vi "array -- bilinear regression 2D -- V2.vi"(7 "action":T2, 9 "fit map IN":map{T1, dbl}(c390), 11 "xyz IN":cluster{"x":dbl[], "y":dbl[], "z":dbl[]}={"x"=[0.0, 0.0, 0.0, -1.0, -1.0, -1.0, 1.0, 1.0, 1.0], "y"=[-1.0, 0.0, 1.0, -1.0, 0.0, 1.0, -1.0, 0.0, 1.0], "z"=[1.0, 0.0, 1.0, 4.0, 1.0, 0.0, 0.0, 1.0, 4.0]}) -> (1 "fit map out":map{T1, dbl}(c390), 3 "xyz OUT":cluster{"x":dbl[], "y":dbl[], "z":dbl[]}={"x"=[0.0, 0.0, 0.0, -1.0, -1.0, -1.0, 1.0, 1.0, 1.0], "y"=[-1.0, 0.0, 1.0, -1.0, 0.0, 1.0, -1.0, 0.0, 1.0], "z"=[1.0, 0.0, 1.0, 4.0, 1.0, 0.0, 0.0, 1.0, 4.0]})   [LabVIEW 2021]
uses:
  array -- fit control .ctl
  array -- bilinear regression 2D.ctl
  <vilib>/Analysis/baseanly.llb/Matrix Type of Inverse Matrix.ctl
  <vilib>/Analysis/baseanly.llb/Real A x B.vi
  <vilib>/Analysis/Matrix/Numeric/Conversions/Array To Matrix - RA2.vi
  <vilib>/Analysis/baseanly.llb/Real Inverse Matrix.vi
  <vilib>/Analysis/Matrix/Numeric/Conversions/Matrix To Array - RM.vi
  <vilib>/Analysis/NI_AALBase.lvlib
  <vilib>/Analysis/Matrix/NI_Matrix.lvlib
panel:
  out "y":dbl[](array[numeric])=[-1.0, 0.0, 1.0, -1.0, 0.0, 1.0, -1.0, 0.0, 1.0]
  out "fit  IN":dbl[](array[numeric])=[1.9, 2.6, 3.3, 1.0, 2.7, 3.9]
  out "fit OUT":dbl[](array[numeric])=[1.0, 1.0, 1.0, 0.0, 0.0, 0.0]
  out "z":dbl[](array[numeric])=[1.0, 0.0, 1.0, 4.0, 1.0, 0.0, 0.0, 1.0, 4.0]
  out "x":dbl[](array[numeric])=[0.0, 0.0, 0.0, -1.0, -1.0, -1.0, 1.0, 1.0, 1.0]
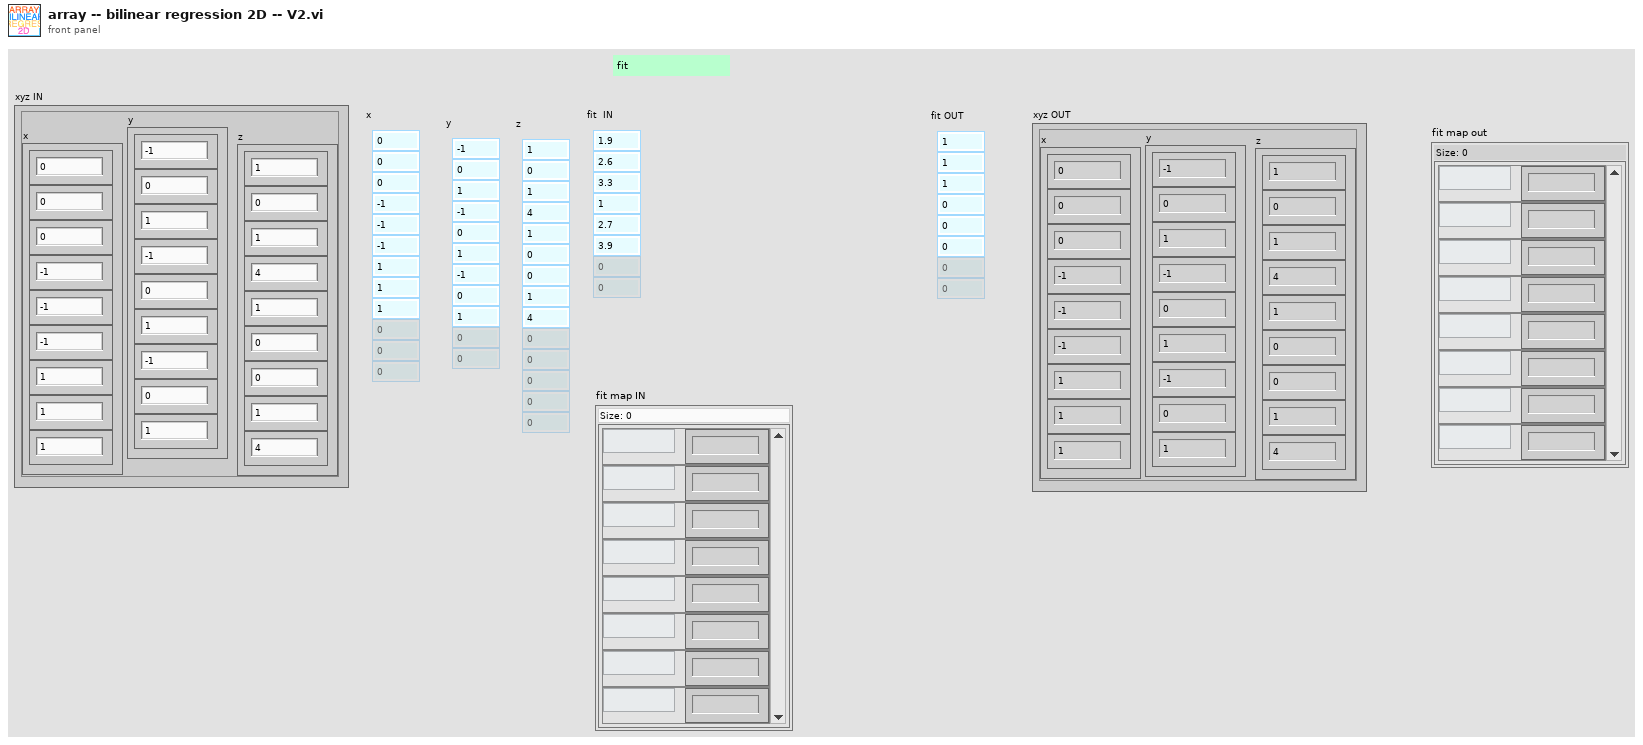
[diagram p1: front panel]
types:
  T1 = typedef "array -- bilinear regression 2D.ctl" = enum16{"1", "x", "y", "xx", "xy", "yy", "xxy", "xyy", "yyy", "xxx", "xxyy", "xyyy", "xxxy", "yyyy", "xxxx", "xxz", "xyz", "yyz", "xz", "yz", "z", "wwz", "ywz", "xwz", "xxxw", "xxyw", "xyyw", "yyyw", "xxww", "xyww", "yyww", "xwww", "ywww", "wwww", "ww", "xw", "yw", "w", "wz"}
  T2 = typedef "array -- fit control .ctl" = enum16{"fit", "calc", "check", "init"}
  T3 = typedef "NI_AALBase.lvlib/Matrix Type of Inverse Matrix.ctl" = enum32{"General", "Positive Definite", "Lower Triangular", "Upper Triangular"}
  T4 = typedef "NI_Matrix.lvlib/RealMatrix.ctl" = dbl[][]
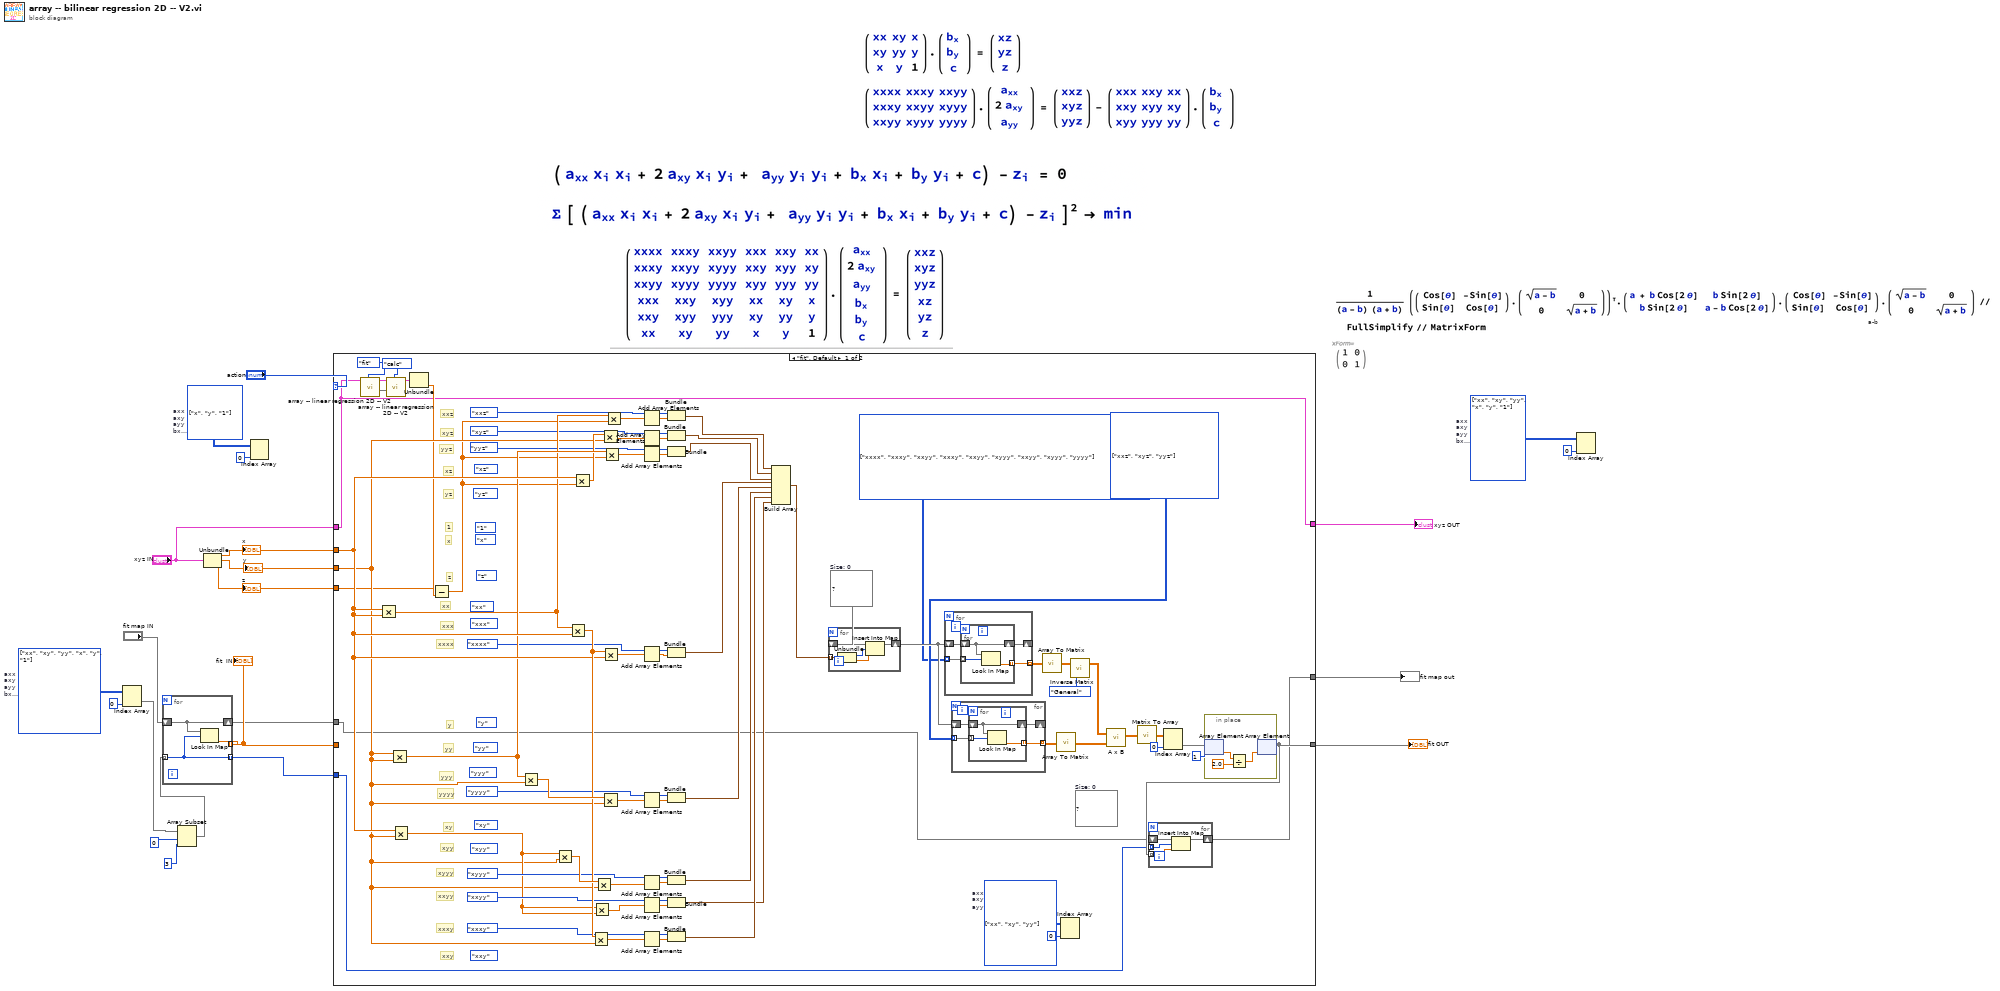
[diagram p0: block diagram]
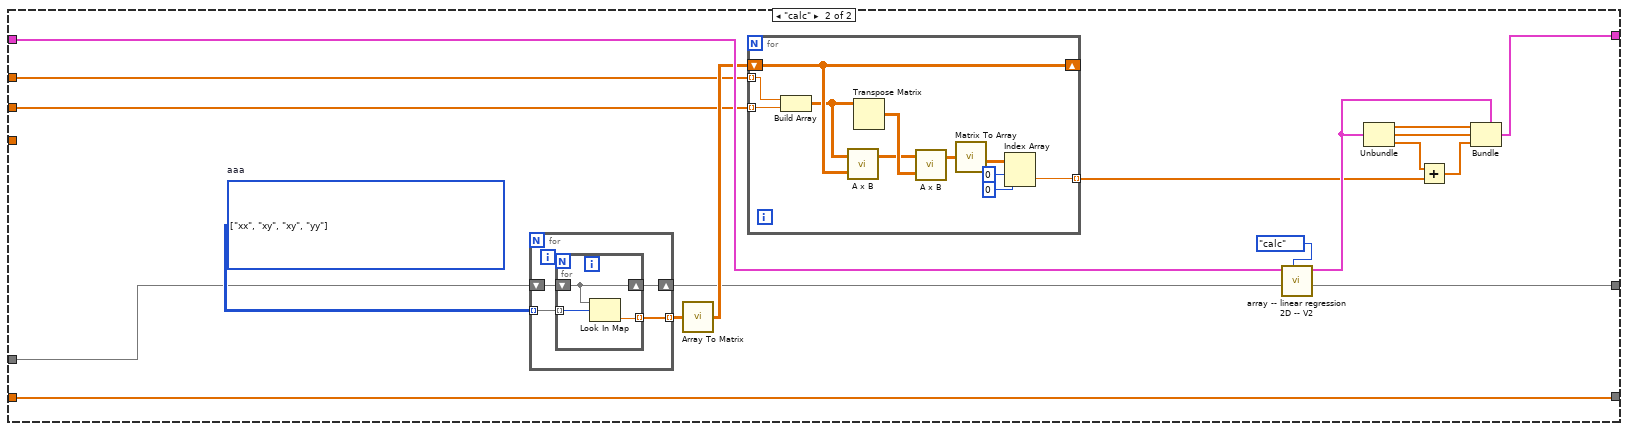
[diagram p2: hidden frame]
diagram:
  w12 = T1[][] [[enum."x"], [enum."y"], [enum."1"]] items=["1", "x", "y", "xx", "xy", "yy", "xxy", "xyy", "yyy", "xxx", "xxyy", "xyyy", "xxxy", "yyyy", "xxxx", "xxz", "xyz", "yyz", "xz", "yz", "z", "wwz", "ywz", "xwz", "xxxw", "xxyw", "xyyw", "yyyw", "xxww", "xyww", "yyww", "xwww", "ywww", "wwww", "ww", "xw", "yw", "w", "wz"]  # axx axy ayy bx by c
  w16 = T1[][] [[enum."xx"], [enum."xy"], [enum."yy"], [enum."x"], [enum."y"], [enum."1"]] items=["1", "x", "y", "xx", "xy", "yy", "xxy", "xyy", "yyy", "xxx", "xxyy", "xyyy", "xxxy", "yyyy", "xxxx", "xxz", "xyz", "yyz", "xz", "yz", "z", "wwz", "ywz", "xwz", "xxxw", "xxyw", "xyyw", "yyyw", "xxww", "xyww", "yyww", "xwww", "ywww", "wwww", "ww", "xw", "yw", "w", "wz"]  # axx axy ayy bx by c
  w18 = T1[][] [[enum."xx"], [enum."xy"], [enum."yy"], [enum."x"], [enum."y"], [enum."1"]] items=["1", "x", "y", "xx", "xy", "yy", "xxy", "xyy", "yyy", "xxx", "xxyy", "xyyy", "xxxy", "yyyy", "xxxx", "xxz", "xyz", "yyz", "xz", "yz", "z", "wwz", "ywz", "xwz", "xxxw", "xxyw", "xyyw", "yyyw", "xxww", "xyww", "yyww", "xwww", "ywww", "wwww", "ww", "xw", "yw", "w", "wz"]  # axx axy ayy bx by c
  # "a-b"
  n1 = Index Array(array=w16, index (col)=0 ("disabled index (col)")) -> (element=w5:T1[])  [unwired: 1 in]
  n2 = Array Subset(array=w5, index=0 ("disabled index (col)"), length=3) -> (w2:T1[])
  n3 = for {
    shift-right: [w24] -> w10
    shift-left: "fit map IN" -> [w24]
    tunnel: w2 -> [w23] mode=indexing
    tunnel: [w25] -> w13 mode=indexing
    tunnel: [w23] -> w1 mode=indexing
    n4 = Look In Map(map=w24, key=w23) -> (value=w25:dbl)  [unwired: 1 in, 1 out]
  }
  "fit  IN" <- w13
  n5 = Unbundle("xyz IN") -> ("x"=w21:dbl[], "y"=w20:dbl[], "z"=w9:dbl[])
  "x" <- w21
  "z" <- w9
  "y" <- w20
  n6 = Index Array(array=w12, index (col)=0 ("disabled index (col)")) -> ()  [unwired: 1 in, 1 out]
  n7 = case shown="\"fit\", Default" "action" {
    tunnel: w9 -> [w33 _]
    tunnel: w21 -> [w84 w124]
    tunnel: [w46 w141] -> w19
    tunnel: w13 -> [_ w141]
    tunnel: w20 -> [w63 w132]
    tunnel: w10 -> [w28 w134]
    tunnel: "xyz IN" -> [w27 w139]
    tunnel: [w29 w138] -> w7
    tunnel: [w27 w125] -> w6
    tunnel: w1 -> [w26 _]
    frame "fit", Default {
      (unwired) map{T1, dbl} {}  # Size: 0
      w31 = T1[][] [[enum."xx"], [enum."xy"], [enum."yy"]] items=["1", "x", "y", "xx", "xy", "yy", "xxy", "xyy", "yyy", "xxx", "xxyy", "xyyy", "xxxy", "yyyy", "xxxx", "xxz", "xyz", "yyz", "xz", "yz", "z", "wwz", "ywz", "xwz", "xxxw", "xxyw", "xyyw", "yyyw", "xxww", "xyww", "yyww", "xwww", "ywww", "wwww", "ww", "xw", "yw", "w", "wz"]  # axx axy ayy
      w44 = T1[][] [[enum."xxz"], [enum."xyz"], [enum."yyz"]] items=["1", "x", "y", "xx", "xy", "yy", "xxy", "xyy", "yyy", "xxx", "xxyy", "xyyy", "xxxy", "yyyy", "xxxx", "xxz", "xyz", "yyz", "xz", "yz", "z", "wwz", "ywz", "xwz", "xxxw", "xxyw", "xyyw", "yyyw", "xxww", "xyww", "yyww", "xwww", "ywww", "wwww", "ww", "xw", "yw", "w", "wz"]
      w43 = T1[][] [[enum."xxxx", enum."xxxy", enum."xxyy"], [enum."xxxy", enum."xxyy", enum."xyyy"], [enum."xxyy", enum."xyyy", enum."yyyy"]] items=["1", "x", "y", "xx", "xy", "yy", "xxy", "xyy", "yyy", "xxx", "xxyy", "xyyy", "xxxy", "yyyy", "xxxx", "xxz", "xyz", "yyz", "xz", "yz", "z", "wwz", "ywz", "xwz", "xxxw", "xxyw", "xyyw", "yyyw", "xxww", "xyww", "yyww", "xwww", "ywww", "wwww", "ww", "xw", "yw", "w", "wz"]
      w47 = map{T1, dbl} {}  # Size: 0
      (unwired) array_--_bilinear_regression_2D."xxy"
      (unwired) array_--_bilinear_regression_2D."xyy"
      (unwired) array_--_bilinear_regression_2D."xy"
      (unwired) array_--_bilinear_regression_2D."yyy"
      (unwired) array_--_bilinear_regression_2D."yy"
      (unwired) array_--_bilinear_regression_2D."y"
      (unwired) array_--_bilinear_regression_2D."xxx"
      (unwired) array_--_bilinear_regression_2D."xx"
      (unwired) array_--_bilinear_regression_2D."x"
      (unwired) array_--_bilinear_regression_2D."1"
      (unwired) array_--_bilinear_regression_2D."z"
      (unwired) array_--_bilinear_regression_2D."yz"
      (unwired) array_--_bilinear_regression_2D."xz"
      # "z"
      # "xxz"
      # "yz"
      # "xz"
      # "yyz"
      # "xyz"
      # "xxy"
      # "xxxy"
      # "xxyy"
      # "xyyy"
      # "xyy"
      # "xy"
      # "yyyy"
      # "yyy"
      # "yy"
      # "y"
      # "1"
      # "xxxx"
      # "xxx"
      # "xx"
      # "x"
      n8 = call "array -- linear regression 2D -- V2.vi"("action"=array_--_fit_control_."fit", "xyz IN"=w27) -> ("fit map out"=w37:map{T1, dbl}, "xyz OUT"=w36:cluster{"x":dbl[], "y":dbl[], "z":dbl[]})  [unwired: 8 in]
      n9 = Multiply(x=w84, y=w84) -> (x*y=w82:dbl[])
      n10 = call "array -- linear regression 2D -- V2.vi"("action"=array_--_fit_control_."calc", "fit map IN"=w37, "xyz IN"=w36) -> ("xyz OUT"=w38:cluster{"x":dbl[], "y":dbl[], "z":dbl[]})  [unwired: 7 in, 1 out]
      n11 = Multiply(x=w63, y=w63) -> (x*y=w83:dbl[])
      n12 = Multiply(x=w84, y=w63) -> (x*y=w66:dbl[])
      n13 = Unbundle(w38) -> ("z"=w39:dbl[])  [unwired: 2 out]
      n14 = Subtract(x=w33, y=w39) -> (x-y=w32:dbl[])
      n15 = Multiply(x=w83, y=w63) -> (x*y=w92:dbl[])
      n16 = Multiply(x=w66, y=w63) -> (x*y=w88:dbl[])
      n17 = Multiply(x=w82, y=w84) -> (x*y=w86:dbl[])
      n18 = Multiply(x=w84, y=w32) -> (x*y=w80:dbl[])
      n19 = Multiply(x=w86, y=w63) -> (x*y=w87:dbl[])
      n20 = Multiply(x=w66, y=w66) -> (x*y=w89:dbl[])
      n21 = Multiply(x=w88, y=w63) -> (x*y=w90:dbl[])
      n22 = Multiply(x=w80, y=w63) -> (x*y=w79:dbl[])
      n23 = Multiply(x=w92, y=w63) -> (x*y=w91:dbl[])
      n24 = Multiply(x=w86, y=w84) -> (x*y=w97:dbl[])
      n25 = Multiply(x=w83, y=w32) -> (x*y=w85:dbl[])
      n26 = Multiply(x=w82, y=w32) -> (x*y=w81:dbl[])
      n27 = Add Array Elements(numeric array=w81) -> (sum=w78:dbl)
      n28 = Add Array Elements(numeric array=w79) -> (sum=w76:dbl)
      n29 = Add Array Elements(numeric array=w85) -> (sum=w73:dbl)
      n30 = Add Array Elements(numeric array=w97) -> (sum=w61:dbl)
      n31 = Add Array Elements(numeric array=w91) -> (sum=w65:dbl)
      n32 = Add Array Elements(numeric array=w90) -> (sum=w68:dbl)
      n33 = Add Array Elements(numeric array=w89) -> (sum=w70:dbl)
      n34 = Add Array Elements(numeric array=w87) -> (sum=w72:dbl)
      n35 = Bundle(array_--_bilinear_regression_2D."xxz", "Numeric"=w78) -> (w40:cluster{T1, "Numeric":dbl})  [unwired: 1 in]
      n36 = Bundle(array_--_bilinear_regression_2D."xyz", "Numeric"=w76) -> (w41:cluster{T1, "Numeric":dbl})  [unwired: 1 in]
      n37 = Bundle(array_--_bilinear_regression_2D."yyz", "Numeric"=w73) -> (w42:cluster{T1, "Numeric":dbl})  [unwired: 1 in]
      n38 = Bundle(array_--_bilinear_regression_2D."xxxx", "Numeric"=w61) -> (w60:cluster{T1, "Numeric":dbl})  [unwired: 1 in]
      n39 = Bundle(array_--_bilinear_regression_2D."yyyy", "Numeric"=w65) -> (w59:cluster{T1, "Numeric":dbl})  [unwired: 1 in]
      n40 = Bundle(array_--_bilinear_regression_2D."xyyy", "Numeric"=w68) -> (w58:cluster{T1, "Numeric":dbl})  [unwired: 1 in]
      n41 = Bundle(array_--_bilinear_regression_2D."xxyy", "Numeric"=w70) -> (w56:cluster{T1, "Numeric":dbl})  [unwired: 1 in]
      n42 = Bundle(array_--_bilinear_regression_2D."xxxy", "Numeric"=w72) -> (w57:cluster{T1, "Numeric":dbl})  [unwired: 1 in]
      n43 = Build Array(w40, w41, w42, w60, w59, w58, w57, w56) -> (w55:cluster{T1, "Numeric":dbl}[])
      n44 = for {
        tunnel: w55 -> [w114] mode=indexing
        shift-right: [w115] -> w45
        shift-left: w47 -> [w116]
        n45 = Unbundle(w114) -> (w113:T1, "Numeric"=w112:dbl)
        n46 = Insert Into Map(map in=w116, key=w113, value=w112) -> (map out=w115:map{T1, dbl})  [unwired: 2 out]
      }
      n47 = for {
        tunnel: w43 -> [w120] mode=indexing
        shift-right: [w118] -> _
        shift-left: w45 -> [w119]
        tunnel: [w117] -> w53 mode=indexing
        n48 = for {
          tunnel: w120 -> [w122] mode=indexing
          shift-right: [w123] -> w118
          shift-left: w119 -> [w123]
          tunnel: [w121] -> w117 mode=indexing
          n49 = Look In Map(map=w123, key=w122) -> (value=w121:dbl)  [unwired: 1 in, 1 out]
        }
      }
      n50 = for {
        shift-right: [w107] -> _
        shift-left: w45 -> [w108]
        tunnel: w44 -> [w106] mode=indexing
        tunnel: [w105] -> w52 mode=indexing
        n51 = for {
          shift-right: [w111] -> w107
          shift-left: w108 -> [w111]
          tunnel: w106 -> [w110] mode=indexing
          tunnel: [w109] -> w105 mode=indexing
          n52 = Look In Map(map=w111, key=w110) -> (value=w109:dbl)  [unwired: 1 in, 1 out]
        }
      }
      n53 = call-poly <vilib>:"Array To Matrix.vi"("Real 2D Array"=w53) -> ("Real Matrix"=w48:T4)
      n54 = call-poly <vilib>:"Array To Matrix.vi"("Real 2D Array"=w52) -> ("Real Matrix"=w51:T4)
      n55 = Index Array(array=w31, index (col)=0 ("disabled index (col)")) -> ()  [unwired: 1 in, 1 out]
      n56 = call-poly <vilib>:"Inverse Matrix.vi"("matrix type"=Matrix_Type_of_Inverse_Matrix."General", "Input Matrix"=w48) -> ("Inverse Matrix"=w96:T4)  [unwired: 1 out]
      n57 = call-poly <vilib>:"A x B.vi"("B"=w51, "A"=w96) -> ("A x B"=w95:T4)  [unwired: 1 out]
      n58 = call-poly <vilib>:"Matrix To Array.vi"("Real Matrix"=w95) -> ("Real 2D Array"=w94:dbl[][])
      n59 = Index Array(array=w94, index (col)=0 ("disabled index (col)")) -> (element=w50:dbl[])  [unwired: 1 in]
      n60 = in-place {
        n61 = in-place-array #1(w50, 1) -> (w104:dbl)
        n62 = Divide(x=w104, y=2.0) -> (x/y=w102:dbl)
        n63 = in-place-array #1(w102) -> (w46:dbl[])  [unwired: 1 out]
      }
      n64 = for {
        shift-right: [w100] -> w29
        shift-left: w28 -> [w101]
        tunnel: w26 -> [w99] mode=indexing
        tunnel: w46 -> [w98] mode=indexing
        n65 = Insert Into Map(map in=w101, key=w99, value=w98) -> (map out=w100:map{T1, dbl})  [unwired: 2 out]
      }
    }
    frame "calc" {
      w136 = T1[][] [[enum."xx", enum."xy"], [enum."xy", enum."yy"]] items=["1", "x", "y", "xx", "xy", "yy", "xxy", "xyy", "yyy", "xxx", "xxyy", "xyyy", "xxxy", "yyyy", "xxxx", "xxz", "xyz", "yyz", "xz", "yz", "z", "wwz", "ywz", "xwz", "xxxw", "xxyw", "xyyw", "yyyw", "xxww", "xyww", "yyww", "xwww", "ywww", "wwww", "ww", "xw", "yw", "w", "wz"]  # aaa
      n66 = for {
        tunnel: w136 -> [w156] mode=indexing
        shift-right: [w154] -> w133
        shift-left: w134 -> [w155]
        tunnel: [w153] -> w137 mode=indexing
        n67 = for {
          tunnel: w156 -> [w158] mode=indexing
          shift-right: [w159] -> w154
          shift-left: w155 -> [w159]
          tunnel: [w157] -> w153 mode=indexing
          n68 = Look In Map(map=w159, key=w158) -> (value=w157:dbl)  [unwired: 1 in, 1 out]
        }
      }
      n69 = call-poly <vilib>:"Array To Matrix.vi"("Real 2D Array"=w137) -> ("Real Matrix"=w135:T4)
      n70 = for {
        tunnel: w132 -> [w151] mode=indexing
        shift-right: [w150] -> _
        shift-left: w135 -> [w150]
        tunnel: [w143] -> w126 mode=indexing
        tunnel: w124 -> [w142] mode=indexing
        n71 = Build Array(w142, w151) -> (w149:T4)
        n72 = call-poly <vilib>:"A x B.vi"("B"=w150, "A"=w149) -> ("A x B"=w147:T4)  [unwired: 1 out]
        n73 = Transpose Matrix(1:w149) -> (0:w148:T4)
        n74 = call-poly <vilib>:"A x B.vi"("B"=w148, "A"=w147) -> ("A x B"=w152:T4)  [unwired: 1 out]
        n75 = call-poly <vilib>:"Matrix To Array.vi"("Real Matrix"=w152) -> ("Real 2D Array"=w146:dbl[][])
        n76 = Index Array(array=w146, index (row)=0, index (col)=0 ("disabled index (col)")) -> (element=w143:dbl)
      }
      n77 = call "array -- linear regression 2D -- V2.vi"("action"=array_--_fit_control_."calc", "fit map IN"=w133, "xyz IN"=w139) -> ("fit map out"=w138:map{T1, dbl}, "xyz OUT"=w127:cluster{"x":dbl[], "y":dbl[], "z":dbl[]})  [unwired: 7 in]
      n78 = Unbundle(w127) -> ("x"=w131:dbl[], "y"=w130:dbl[], "z"=w129:dbl[])
      n79 = Add(x=w129, y=w126) -> (x+y=w128:dbl[])
      n80 = Bundle(cluster=w127, "x"=w131, "y"=w130, "z"=w128) -> (w125:cluster{"x":dbl[], "y":dbl[], "z":dbl[]})
    }
  }
  "fit OUT" <- w19
  "fit map out" <- w7
  "xyz OUT" <- w6
  n81 = Index Array(array=w18, index (col)=0 ("disabled index (col)")) -> ()  [unwired: 1 in, 1 out]
